vi "Sort_array_to_case.vi"(1 "Array to sort":u16[](array[numeric]), 2 "Equi spaced data Only?":bool) -> (0 "Sorted Array":i32[](array[numeric]))   [LabVIEW 2010]
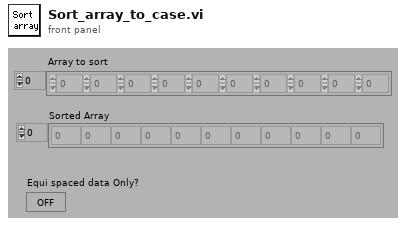
[diagram p1: front panel]
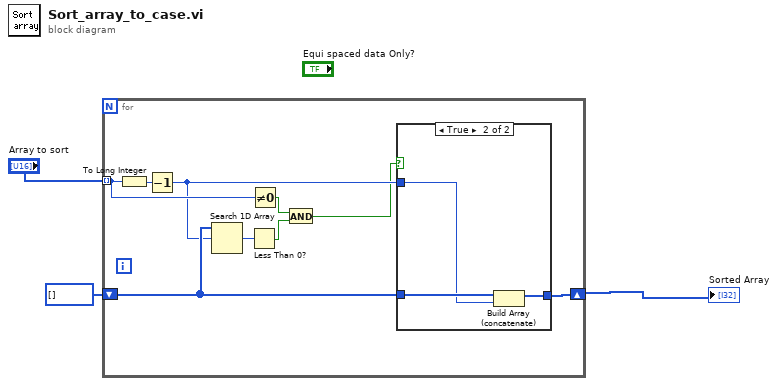
[diagram p0: block diagram]
diagram:
  n1 = for {
    tunnel: "Array to sort" -> [w9] mode=indexing
    shift-right: [w11] -> w1
    shift-left: i32[] [] -> [w12]
    n2 = To Long Integer(number=w9) -> (32bit integer=w6:i32)
    n3 = Decrement(x=w6) -> (x-1=w5:i32)
    n4 = Search 1D Array(1D array=w12, element=w5) -> (index of element=w10:i32)  [unwired: 1 out]
    n5 = Less Than 0?(x=w10) -> (x < 0?=w8:bool)
    n6 = Not Equal To 0?(x=w9) -> (x != 0?=w7:bool)
    n7 = And(x=w7, y=w8) -> (x .and. y?=w4:bool)
    n8 = case shown="True" w4 {
      tunnel: w12 -> [w13 w16]
      tunnel: w5 -> [_ w14]
      tunnel: [w13 w15] -> w11
      frame False {
      }
      frame True {
        n9 = Build Array (concatenate)(w16, w14) -> (w15:i32[])
      }
    }
  }
  "Sorted Array" <- w1
